vi "Digital IO UI.vi"() -> ()   [LabVIEW 2025, in "Digital IO.lvlib" / "Digital IO Instrument.lvclass"]
doc: "Copyright 2017 National Instruments Corporation\n\nLicensed under the Apache License, Version 2.0 (the \"License\"); you may not use this file except in compliance with the License. You may obtain a copy of the License at http://www.apache.org/licenses/LICENSE-2.0\nUnless required by applicable law or agreed to in writing, software distributed under the License is distributed on an \"AS IS\" BASIS, WITHOUT WARRANTIES OR CONDITIONS OF ANY KIND, either express or implied. See the License for the specific language governing permissions and limitations under the License."
uses:
  Digital IO Instrument.lvclass
  Users/Public/Documents/Sandia National Labs/TSS Plugin/CEF.lvlibp/Node/NodeRef.ctl
  Users/Public/Documents/Sandia National Labs/TSS Plugin/CEF.lvlibp/Node/CEF_Node.lvclass
  Users/Public/Documents/Sandia National Labs/TSS Plugin/CEF.lvlibp/Node/mainQref.ctl
  Users/Public/Documents/Sandia National Labs/TSS Plugin/CEF.lvlibp/Node/UserEventRef.ctl
  Users/Public/Documents/Sandia National Labs/TSS Plugin/Abstract Engine.lvlibp/Plugin/Abstract/Instrument configuration/Default Instrument.ctl
  Digital IO Instrument.lvclass/Digital IO Instrument.ctl
  <vilib>/Utility/error.llb/Trim Whitespace One-Sided.vi
  Users/Public/Documents/Sandia National Labs/TSS Plugin/Abstract Engine.lvlibp/Plugin/Abstract/Instrument configuration/Read Instrument Setting.vi
  Users/Public/Documents/Sandia National Labs/TSS Plugin/Abstract Engine.lvlibp/Plugin/Abstract/Instrument configuration/Write Instrument Setting.vi
  C:/Users/Public/Documents/Sandia National Labs/TSS Plugin/Abstract Engine.lvlibp/Plugin/Abstract/Abstract Instrument/Abstract Instrument.lvclass
  C:/Users/Public/Documents/Sandia National Labs/TSS Plugin/CEF.lvlibp/serializable node/CEF_serializable node.lvclass
  C:/Users/Public/Documents/Sandia National Labs/TSS Plugin/CEF.lvlibp/Node/CEF_Node.lvclass
  C:/Users/Public/Documents/Sandia National Labs/TSS Plugin/Interface.lvlibp/Analog Input/AI.lvclass
  C:/Working copy/tss/Plugin/Engines/Digital IO/Digital IO Instrument/Digital IO Instrument.lvclass
  C:/Users/Public/Documents/Sandia National Labs/TSS Plugin/Interface.lvlibp/Digital Input/DI.lvclass
  C:/Users/Public/Documents/Sandia National Labs/TSS Plugin/Interface.lvlibp/Digital Output/DO.lvclass
  Users/Public/Documents/Sandia National Labs/TSS Plugin/Abstract Engine.lvlibp/Plugin/Abstract/Instrument configuration/Instrument configuration.lvclass
panel:
  in  "Digital IO":T1={"Type"="None", "Address"="None", "SW Alias"="None", "Description"="* Type = Class", "Enabled"=TRUE}
  in  "user event":T2
  in  "main queue":T3
  in  "node ref":T4
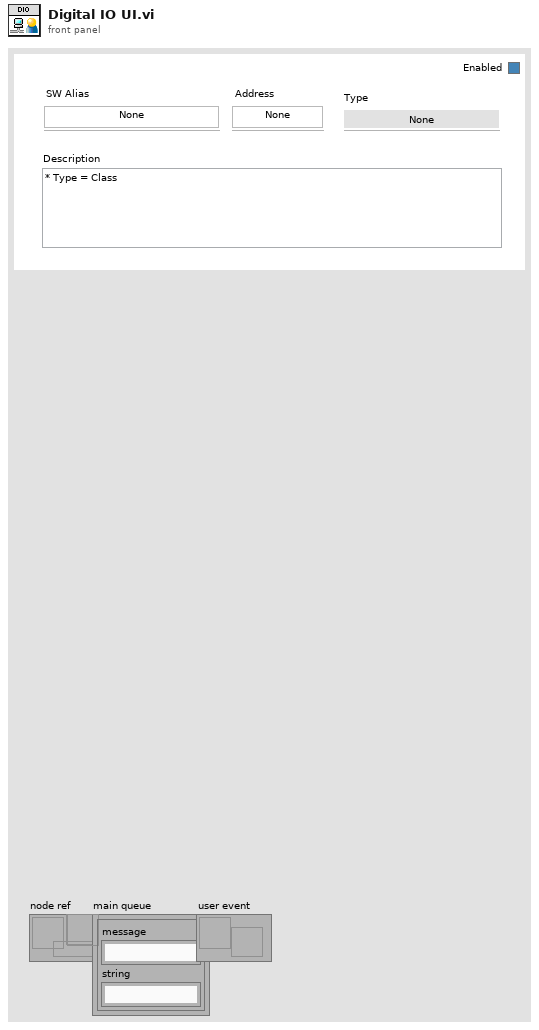
[diagram p1: front panel]
types:
  T1 = typedef "Abstract Engine.lvlibp/Instrument configuration.lvclass/Default Instrument.ctl" = cluster{"Type":string, "Address":string, "SW Alias":string, "Description":string, "Enabled":bool}
  T2 = typedef "CEF.lvlibp/CEF_Node.lvclass/UserEventRef.ctl" = refnum<user-event>
  T3 = typedef "CEF.lvlibp/CEF_Node.lvclass/mainQref.ctl" = refnum<queue>
  T4 = typedef "CEF.lvlibp/CEF_Node.lvclass/NodeRef.ctl" = refnum<data-value>
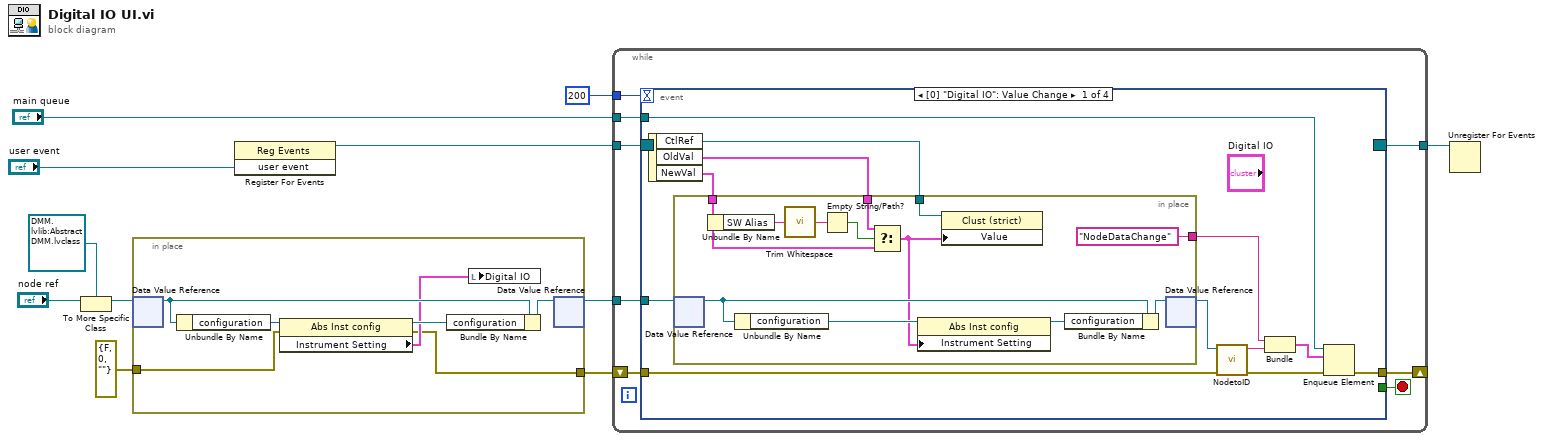
[diagram p0: block diagram]
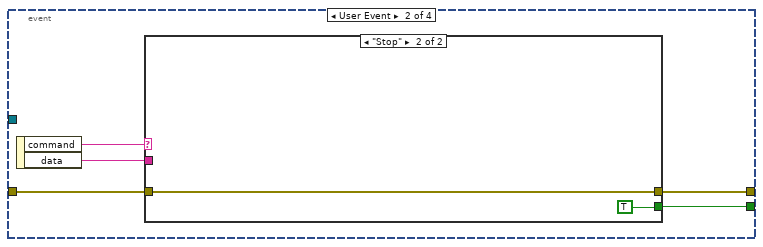
[diagram p2: hidden frame]
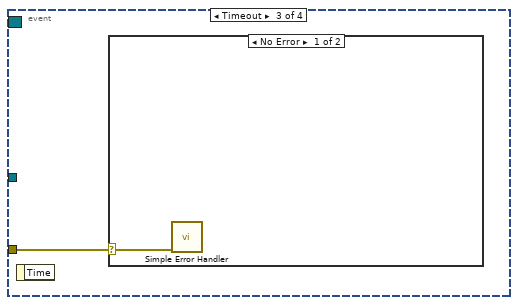
[diagram p4: hidden frame]
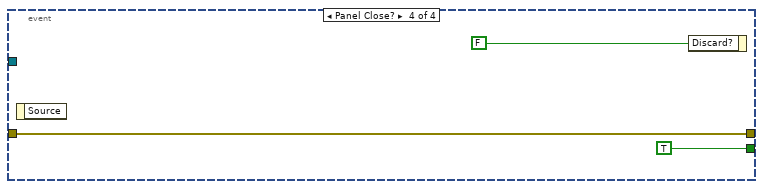
[diagram p6: hidden frame]
diagram:
  n1 = To More Specific Class(target class=refnum<data-value> refnum ("data value reference"), reference="node ref") -> (specific class reference=w8:refnum<data-value>)  [unwired: 1 in, 1 out]
  n2 = in-place {
    in-place-border: errorcluster {"status"=FALSE, "code"=0, "source"=""} ("error out") -> [w13]
    in-place-border: [w12] -> w2
    # "Initialize the front panel controls when loaded"
    n3 = in-place-dvr #1(w8) -> (w17:refnum<class "Digital IO Instrument.lvclass">)  [unwired: 1 out]
    n4 = Unbundle By Name(w17) -> ("configuration"=w18:refnum<class "Instrument configuration.lvclass">)
    n5 = property class="Abs Inst config"(reference=w18, error in=w13) -> (reference out=w16:refnum<class "Instrument configuration.lvclass">, error out=w12:errorcluster, "Instrument Setting"=w14:T1)
    n6 = Bundle By Name(cluster=w17, "configuration"=w16) -> (w15:refnum<class "Digital IO Instrument.lvclass">)
    n7 = local write "Digital IO"(w14) -> ()
    n8 = in-place-dvr #1(w15) -> (w7:refnum<data-value>)  [unwired: 1 out]
  }
  n9 = register-events("user event") -> (reference out=w11:refnum<event-registration>)  [unwired: 2 in, 1 out]
  n10 = while {
    tunnel: w7 -> [w26]
    tunnel: w11 -> [w25]
    tunnel: [w24] -> w10
    tunnel: "main queue" -> [w20]
    shift-right: [w21] -> _
    shift-left: w2 -> [w22]
    tunnel: 200 -> [w19]
    stop <- w23 stop-if-true
    n11 = event shown="[0] \"Digital IO\": Value Change" {
      selector: w25 -> [_ _ _ _]
      dyn-events: [_ _ _ _] -> w24
      timeout: w19 -> [_ _ _ _]
      tunnel: w26 -> [w36 _ _ _]
      tunnel: [_ w55 _ TRUE] -> w23
      tunnel: [w37 w51 _ w62] -> w21
      tunnel: w22 -> [w28 w53 w59 w62]
      tunnel: w20 -> [w38 _ _ _]
      event Value Change {
        n12 = event-data() -> ("CtlRef"=w32:refnum<vi>, "OldVal"=w33:T1, "NewVal"=w34:T1)  [unwired: 1 in]
        n13 = in-place {
          in-place-border: w34 -> [w45]
          in-place-border: w33 -> [w43]
          in-place-border: w32 -> [w42]
          in-place-border: ["NodeDataChange" ("Message Name")] -> w31
          n14 = in-place-dvr #2(w36) -> (w50:refnum<class "Digital IO Instrument.lvclass">)  [unwired: 1 out]
          n15 = Unbundle By Name(w45) -> ("SW Alias"=w46:string)
          n16 = Unbundle By Name(w50) -> ("configuration"=w49:refnum<class "Instrument configuration.lvclass">)
          n17 = call <vilib>:"Trim Whitespace.vi"("string"=w46) -> ("trimmed string"=w41:string)  [unwired: 1 in]
          n18 = Empty String/Path?(string/path=w41) -> (empty?=w44:bool)
          n19 = Select(t=w43, s=w44, f=w45) -> (s? t:f=w40:T1)
          n20 = property class="Abs Inst config"(reference=w49, "Instrument Setting"=w40) -> (reference out=w47:refnum<class "Instrument configuration.lvclass">)  [unwired: 1 in, 1 out]
          n21 = property class="Clust (strict)"(reference=w42, "Value"=w40) -> ()  [unwired: 1 in, 2 out]
          n22 = Bundle By Name(cluster=w50, "configuration"=w47) -> (w48:refnum<class "Digital IO Instrument.lvclass">)
          n23 = in-place-dvr #2(w48) -> (w35:refnum<data-value>)  [unwired: 1 out]
        }
        n24 = call "NodetoID.vi"("error in"=w28, "node ref"=w35) -> ("error out"=w27:errorcluster, "ID"=w30:string)  [unwired: 8 in]
        n25 = Bundle("Message Name"=w31, "ID"=w30) -> (w29:cluster{"Message Name":string, "ID":string})  [unwired: 1 in]
        n26 = Enqueue Element(queue=w38, element=w29, error in (no error)=w27) -> (error out=w37:errorcluster)  [unwired: 1 in, 2 out]
      }
      event User Event {
        n27 = event-data() -> ("command"=w52:string, "data"=w54:string)  [unwired: 1 in]
        n28 = case shown="\"Stop\"" w52 {
          tunnel: [_ TRUE] -> w55
          tunnel: w54 -> [_ _]
          tunnel: w53 -> [w56 w57]
          tunnel: [w56 w57] -> w51
          frame Default {
          }
          frame "Stop" {
          }
        }
      }
      event Timeout {
        n29 = event-data() -> ()  [unwired: 1 in, 1 out]
        n30 = case shown="No Error" w59 {
          selector: w59 -> [w60 _]
          frame No Error {
            n31 = call <vilib>:"Simple Error Handler.vi"("error in (no error)"=w60) -> ()  [unwired: 4 in, 5 out]
          }
          frame Error {
          }
        }
      }
      event Panel Close? {
        n32 = event-data() -> ()  [unwired: 1 in, 1 out]
        n33 = event-data("Discard?"=FALSE) -> ()  [unwired: 1 in, 1 out]
      }
    }
  }
  n34 = Unregister For Events(event registration refnum=w10) -> ()  [unwired: 1 in, 1 out]
